vi "禹山溶解氧_获取温度和测量值.vi"(5 "大气压补偿":dbl=1.0, 7 "盐度补偿":dbl, 8 "error in (no error)":errorcluster caption="错误输入（无错误）", 11 "MB session in":refnum<class "MB_Master.lvclass">) -> (0 "error out":errorcluster caption="错误输出", 2 "输出值":cluster{"温度测量值":sgl, "DO%":sgl, "DOmg/L":sgl}, 3 "MB session out":refnum<class "MB_Master.lvclass">)   [LabVIEW 2016, in "斯坦道多参数.lvlib"]
uses:
  <vilib>/Plasmionique/MB Master/MB_Master/MB_Master.lvclass
  <vilib>/Plasmionique/MB Master/MB Master.lvlib
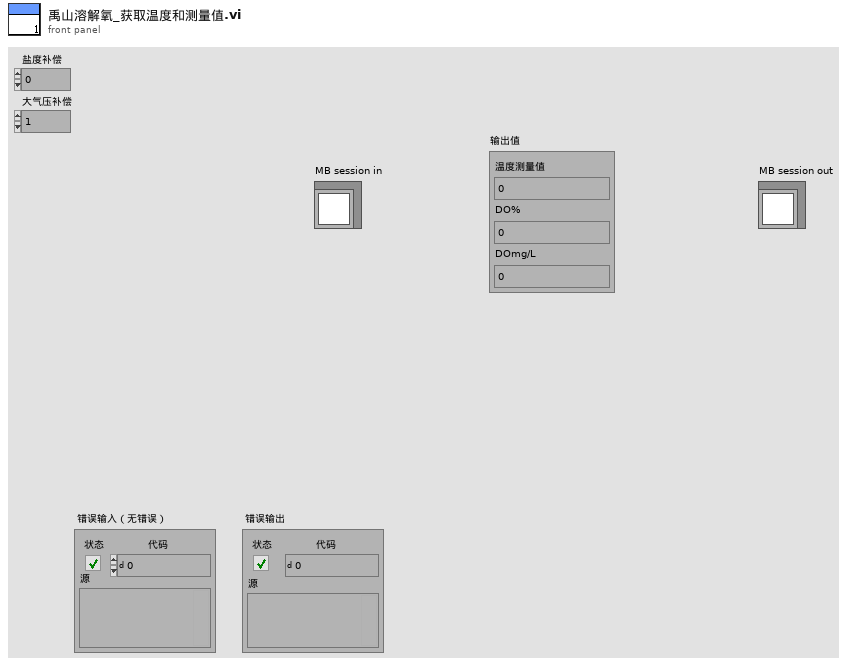
[diagram p1: front panel]
types:
  T1 = cluster{"pH":u32, "DO":u32, "Cond":u32, "Turb":u32, "叶绿素a":u32, "藻密度":u32, "ORP":u32}
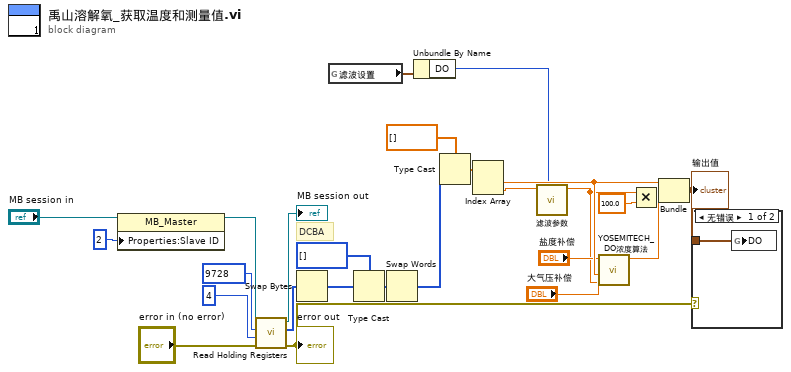
[diagram p0: block diagram]
diagram:
  # "DCBA"
  n1 = property class="MB_Master"(reference="MB session in", "Properties:Slave ID"=u16 2 ("y")) -> (reference out=w18:refnum<class "MB_Master.lvclass">)  [unwired: 1 in, 1 out]
  n2 = call <vilib>:"Read Holding Registers.vi"("error in (no error)"="error in (no error)", "quantity"=u16 4, "starting address"=u16 9728, "MB session in"=w18) -> ("error out"=w8:errorcluster, "Registers"=w16:u16[], "MB session out"=→"MB session out":refnum<class "MB_Master.lvclass">)  [unwired: 5 in]
  "error out" <- w8
  n3 = Swap Bytes(anything=w16) -> (byte swapped=w15:u16[])
  n4 = global read "断电保存变量.vi" "滤波设置"() -> (w2:T1)
  n5 = Type Cast(type=u32[] [] ("数组 2"), x=w15) -> (*(type *) &x=w22:u32[])
  n6 = Swap Words(1:w22) -> (0:w24:u32[])
  n7 = Unbundle By Name(w2) -> ("DO"=w1:u32)
  n8 = Type Cast(type=sgl[] [] ("数组 2"), x=w24) -> (*(type *) &x=w20:sgl[])
  n9 = Index Array(array=w20) -> (element #1=w14:sgl, element #2=w4:sgl)  [unwired: 2 in]
  n10 = call "滤波参数.vi"("滤波次数"=w1, "x"=w4) -> ("mode"=w3:dbl)  [unwired: 9 in]
  n11 = call "YOSEMITECH_DO浓度算法.vi"("溶解氧饱和度值"=w3, "水温"=w14, "大气压补偿"="大气压补偿", "盐度补偿"="盐度补偿") -> ("DataDo_mgL"=w13:dbl)  [unwired: 7 in]
  n12 = Multiply(x=w3, y=sgl 100.0) -> (x*y=w10:dbl)
  n13 = Bundle("数值"=w14, w10, "DataDo_mgL"=w13) -> (w7:cluster{"数值":sgl, dbl, "DataDo_mgL":dbl})  [unwired: 1 in]
  "输出值" <- w7
  n14 = case shown="无错误" w8 {
    tunnel: w7 -> [w27 _]
    frame No Error {
      n15 = global write "禹山过程全局变量.vi" "DO"(w27) -> ()
    }
    frame Error {
    }
  }
